vi "Save To Wav.vi"(0 "Boolean in":refnum<vi>, 1 "output waveform":waveform(dbl), 2 "Bool Refnum":refnum<vi>, 3 "Enum in":enum16{"idle", "open", "write", "save"}(ring), 5 "reference in":refnum<vi>, 9 "Array in":waveform(dbl)[](array[waveform]), 11 "error in (no error)":errorcluster, 12 "Start Recording":bool, 14 "Save To File in":bool) -> (4 "Boolean":bool, 6 "Array out":waveform(dbl)[](array[waveform]), 10 "Enum out":enum16{"idle", "open", "write", "save"}(ring), 15 "error out":errorcluster)   [LabVIEW 2024]
uses:
  <vilib>/sound2/lvsound2.llb/Sound File Write Open.vi
  <vilib>/sound2/lvsound2.llb/Sound File Write (DBL).vi
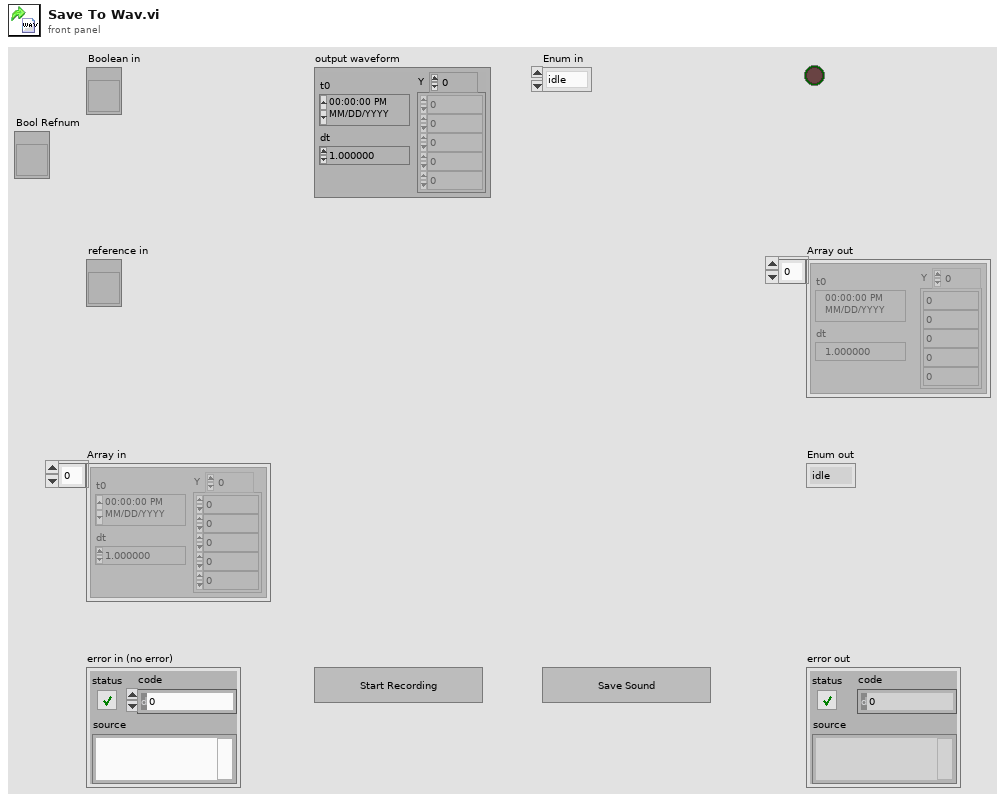
[diagram p1: front panel]
types:
  T1 = enum8{"Enabled", "Disabled", "Disabled and Grayed Out"}
  T2 = typedef "Sound File Refnum.ctl" = refnum<file>
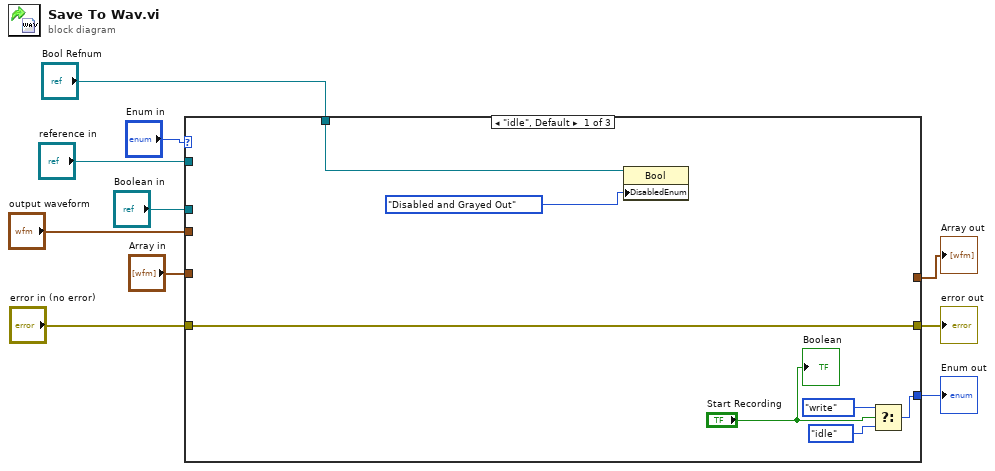
[diagram p0: block diagram]
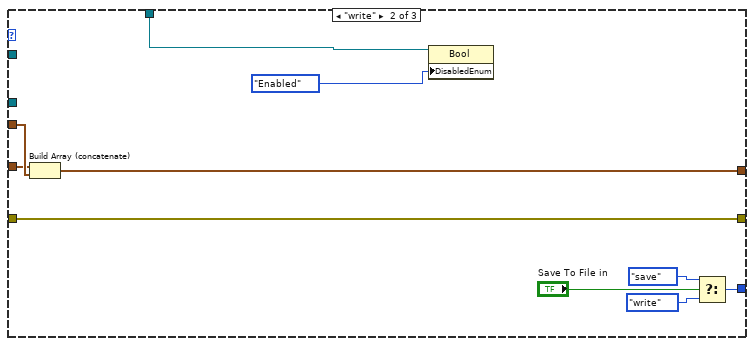
[diagram p2: hidden frame]
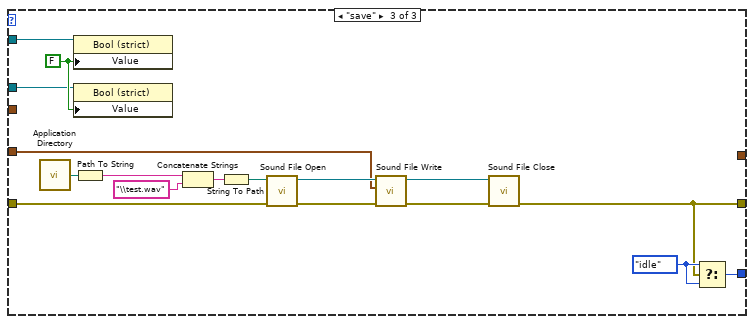
[diagram p3: hidden frame]
diagram:
  n1 = case shown="\"idle\", Default" "Enum in" {
    tunnel: "output waveform" -> [_ w27 _]
    tunnel: [w17 w21 w36] -> w4
    tunnel: "error in (no error)" -> [w17 w21 w37]
    tunnel: [w15 w23 w43] -> w5
    tunnel: [_ w22 _] -> w7
    tunnel: "Array in" -> [_ w20 w31]
    tunnel: "Boolean in" -> [_ _ w29]
    tunnel: "reference in" -> [_ _ w28]
    tunnel: "Bool Refnum" -> [w12 w19 _]
    frame "idle", Default {
      n2 = property on="Property Node" class="Bool"(reference=w12, "DisabledEnum"=T1."Disabled and Grayed Out" ("Disabled")) -> ()  [unwired: 1 in, 2 out]
      n3 = Select(t=enum16{"idle", "open", "write", "save"}."write", s="Start Recording", f=enum16{"idle", "open", "write", "save"}."idle") -> (s? t:f=w15:enum16{"idle", "open", "write", "save"})
      "Boolean" <- "Start Recording"
    }
    frame "write" {
      n4 = Build Array (concatenate)(w20, w27) -> (w22:waveform(dbl)[])
      n5 = property on="Property Node" class="Bool"(reference=w19, "DisabledEnum"=T1."Enabled" ("Disabled")) -> ()  [unwired: 1 in, 2 out]
      n6 = Select(t=enum16{"idle", "open", "write", "save"}."save", s="Save To File in", f=enum16{"idle", "open", "write", "save"}."write") -> (s? t:f=w23:enum16{"idle", "open", "write", "save"})
    }
    frame "save" {
      w30 = FALSE ("Start Recording")
      w44 = enum16{"idle", "open", "write", "save"}."idle"
      n7 = call <vilib>:"Application Directory.vi"() -> ("Application Directory"=w39:path)
      n8 = property class="Bool (strict)"(reference=w28, "Value"=w30) -> ()  [unwired: 1 in, 2 out]
      n9 = property class="Bool (strict)"(reference=w29, "Value"=w30) -> ()  [unwired: 1 in, 2 out]
      n10 = Path To String(path=w39) -> (string=w40:string)
      n11 = Concatenate Strings(w40, "\\test.wav" ("string")) -> (w42:string)
      n12 = String To Path(string=w42) -> (path=w41:path)
      n13 = call-poly <vilib>:"Sound File Open.vi"("error in (no error)"=w37, "path"=w41) -> ("error out"=w35:errorcluster, "sound file refnum"=w32:T2)  [unwired: 1 in, 7 out]
      n14 = call-poly <vilib>:"Sound File Write.vi"("error in (no error)"=w35, "data"=w31, "sound file refnum"=w32) -> ("error out"=w34:errorcluster, "sound file refnum out"=w33:T2)  [unwired: 7 out]
      n15 = call <vilib>:"Sound File Close.vi"("error in (no error)"=w34, "sound file refnum"=w33) -> ("error out"=w36:errorcluster)  [unwired: 9 out]
      n16 = Select(t=w44, s=w36, f=w44) -> (s? t:f=w43:enum16{"idle", "open", "write", "save"})
    }
  }
  "Array out" <- w7
  "Enum out" <- w5
  "error out" <- w4
